vi "SimplePyScriptTests.vi"() -> ()   [LabVIEW 2022 SP3]
uses:
  <vilib>/Utility/error.llb/Trim Whitespace One-Sided.vi
panel:
  out "TotalResponseOutLength":i32
  out "TotalResponseOut":string
  in  "Content Type":string
  in  "Response First Line + CRLF":string="HTTP/1.1 200 OK\r\n"
  in  "Response Header Template":string="User-Agent: LabVIEW WebServer/0.1\nDate: RESPONSE_DATE\nExpires: RESPONSE_DATE\nIgnore-Buffer: xXxBUFFERxXx\nContent-Type: CONTENT_TYPE\nContent-Length: RESPONSE_LENGTH\nConnection: keep-alive"
  in  "ResponseBody":string
  out "Header":string
  out "Body":string
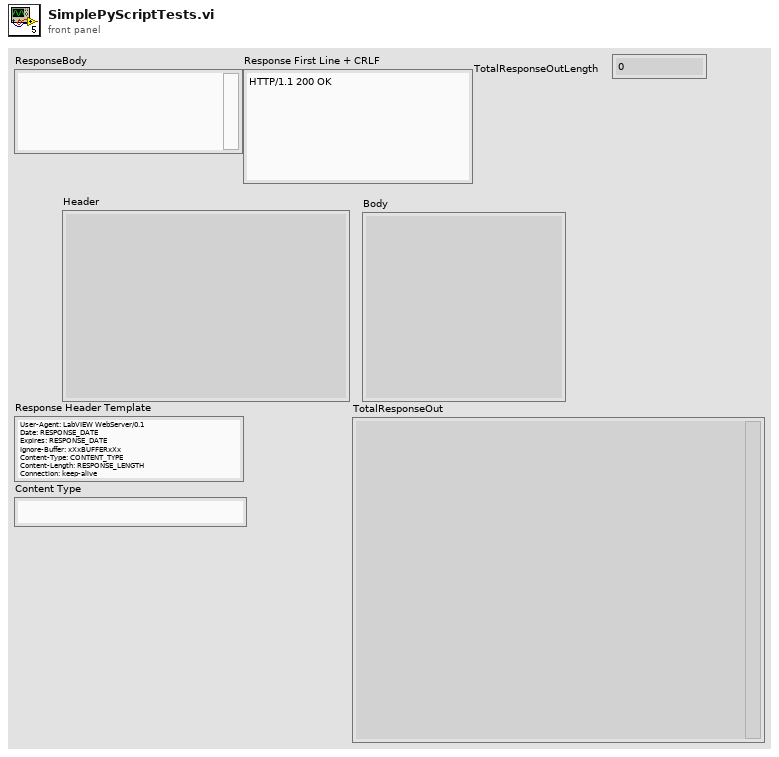
[diagram p1: front panel]
types:
  T1 = enum16{"Standard", "Buffered", "CRLF", "Immediate"}
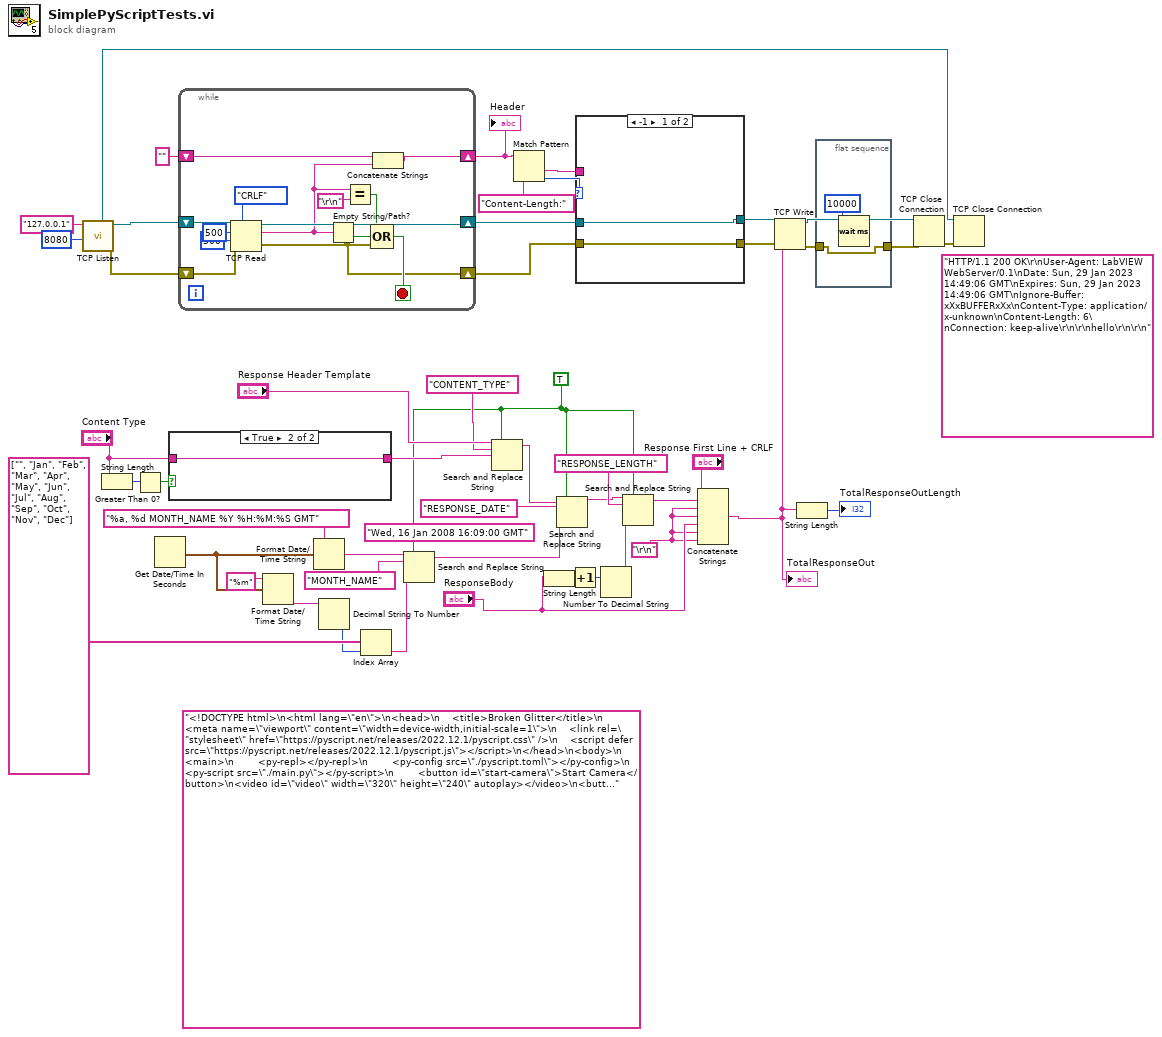
[diagram p0: block diagram]
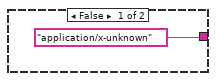
[diagram p2: hidden frame]
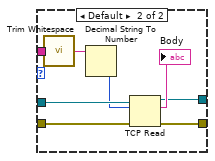
[diagram p3: hidden frame]
diagram:
  w1 = "\r\n"
  (unwired) "<!DOCTYPE html>\n<html lang=\"en\">\n<head>\n    <title>Broken Glitter</title>\n    <meta name=\"viewport\" content=\"width=device-width,initial-scale=1\">\n    <link rel=\"stylesheet\" href=\"https://pyscript.net/releases/2022.12.1/pyscript.css\" />\n    <script defer src=\"https://pyscript.net/releases/2022.12.1/pyscript.js\"></script>\n</head>\n<body>\n    <main>\n        <py-repl></py-repl>\n        <py-config src=\"./pyscript.toml\"></py-config>\n        <py-script src=\"./main.py\"></py-script>\n        <button id=\"start-camera\">Start Camera</button>\n<video id=\"video\" width=\"320\" height=\"240\" autoplay></video>\n<button id=\"click-photo\">Click Photo</button>\n<canvas id=\"canvas\" width=\"320\" height=\"240\"></canvas>\n\n    </main>\n</body>\n</html>" ("data in")
  w7 = TRUE ("replace all? (F)")
  (unwired) "Wed, 16 Jan 2008 16:09:00 GMT" ("replace string (\"\")")
  (unwired) "HTTP/1.1 200 OK\r\nUser-Agent: LabVIEW WebServer/0.1\nDate: Sun, 29 Jan 2023 14:49:06 GMT\nExpires: Sun, 29 Jan 2023 14:49:06 GMT\nIgnore-Buffer: xXxBUFFERxXx\nContent-Type: application/x-unknown\nContent-Length: 6\nConnection: keep-alive\r\n\r\nhello\r\n\r\n" ("data in")
  n1 = call <vilib>:"TCP Listen.vi"("port"=u16 8080, "service name"="127.0.0.1") -> ("error out"=w44:errorcluster, "connection ID"=w46:refnum<k5>, "listener ID"=w32:refnum<k5>)  [unwired: 5 in, 2 out]
  n2 = String Length(string="Content Type") -> (length=w20:i32)
  n3 = Greater Than 0?(x=w20) -> (x > 0?=w21:bool)
  n4 = Get Date/Time In Seconds() -> (seconds since 1Jan1904=w16:timestamp)
  n5 = case shown="True" w21 {
    tunnel: "Content Type" -> [_ w50]
    tunnel: ["application/x-unknown" w50] -> w18
    frame False {
    }
    frame True {
    }
  }
  n6 = while {
    shift-right: [w54] -> w40
    shift-left: w46 -> [w64]
    shift-right: [w59] -> w43
    shift-left: "" -> [w60]
    shift-right: [w55] -> w39
    shift-left: w44 -> [w58]
    stop <- w56 stop-if-true
    n7 = TCP Read(connection ID=w64, bytes to read=500, error in (no error)=w58, 7:T1."CRLF" ("mode (standard)"), 9:500 ("timeout ms (25000)")) -> (connection ID out=w54:refnum<k5>, data out=w53:string, error out=w55:errorcluster)
    n8 = Empty String/Path?(string/path=w53) -> (empty?=w57:bool)
    n9 = Equal?(x=w53, y="\r\n") -> (x = y?=w51:bool)
    n10 = Compound Arithmetic op=OR(w51, w57, w55) -> (w56:bool)
    n11 = Concatenate Strings(w60, w53) -> (w59:string)
  }
  "Header" <- w43
  n12 = Format Date/Time String(time format string (%c)="%m", seconds (now)=w16) -> (date/time string=w14:string)  [unwired: 1 in]
  n13 = Format Date/Time String(time format string (%c)="%a, %d MONTH_NAME %Y %H:%M:%S GMT", seconds (now)=w16) -> (date/time string=w11:string)  [unwired: 1 in]
  n14 = Decimal String To Number(string=w14) -> (number=w12:i32)  [unwired: 3 out]
  n15 = Index Array(array=string[] ["", "Jan", "Feb", "Mar", "Apr", "May", "Jun", "Jul", "Aug", "Sep", "Oct", "Nov", "Dec"], index=w12) -> (element=w9:string)
  n16 = Search and Replace String(replace all?=w7, input string=w11, search string="MONTH_NAME", replace string=w9) -> (result string=w8:string)  [unwired: 4 in, 3 out]
  n17 = Search and Replace String(replace all?=w7, input string="Response Header Template", search string="CONTENT_TYPE", replace string=w18) -> (result string=w28:string)  [unwired: 4 in, 3 out]
  n18 = Match Pattern(string=w43, regular expression="Content-Length:") -> (after substring=w41:string, offset past match=w31:i32)  [unwired: 1 in, 2 out]
  n19 = String Length(string="ResponseBody") -> (length=w5:i32)
  n20 = Search and Replace String(replace all?=w7, input string=w28, search string="RESPONSE_DATE", replace string=w8) -> (result string=w23:string)  [unwired: 4 in, 3 out]
  n21 = Increment(x=w5) -> (x+1=w4:i32)
  n22 = case shown="-1" w31 {
    tunnel: w41 -> [_ w74]
    tunnel: w40 -> [w66 w72]
    tunnel: w39 -> [w65 w70]
    tunnel: [w66 w68] -> w38
    tunnel: [w65 w67] -> w37
    frame -1 {
    }
    frame Default {
      n23 = call <vilib>:"Trim Whitespace.vi"("string"=w74) -> ("trimmed string"=w73:string)  [unwired: 1 in]
      n24 = Decimal String To Number(string=w73) -> (number=w71:i32)  [unwired: 2 in, 1 out]
      n25 = TCP Read(connection ID=w72, bytes to read=w71, error in (no error)=w70) -> (connection ID out=w68:refnum<k5>, data out=→"Body":string, error out=w67:errorcluster)  [unwired: 2 in]
    }
  }
  n26 = Number To Decimal String(number=w4) -> (decimal integer string=w25:string)  [unwired: 1 out]
  n27 = Search and Replace String(replace all?=w7, input string=w23, search string="RESPONSE_LENGTH", replace string=w25) -> (result string=w26:string)  [unwired: 4 in, 3 out]
  n28 = Concatenate Strings("Response First Line + CRLF", w26, w1, w1, "ResponseBody", w1, w1) -> (w2:string)
  "TotalResponseOut" <- w2
  n29 = TCP Write(connection ID=w38, data in=w2, error in (no error)=w37) -> (connection ID out=w34:refnum<k5>, error out=w36:errorcluster)  [unwired: 1 in, 1 out]
  n30 = String Length(string=w2) -> (length=→"TotalResponseOutLength":i32)
  n31 = flat-sequence {
    tunnel: [w75] -> w35
    tunnel: w36 -> [w75]
    frame #0 {
      n32 = Wait (ms)(milliseconds to wait=u32 10000) -> ()  [unwired: 1 out]
    }
  }
  n33 = TCP Close Connection(connection ID=w34, error in (no error)=w35) -> (error out=w33:errorcluster)  [unwired: 1 in, 1 out]
  n34 = TCP Close Connection(connection ID=w32, error in (no error)=w33) -> ()  [unwired: 1 in, 2 out]
